vi "ADCP_Raw_Bytes_To_Data_Packet.vi"(8 "error in (no error)":errorcluster, 9 "Raw Packet":u8[](array[numeric]), 10 "Data Packet In":T2, 11 "ADCP in":refnum<class "ADCP.lvclass">) -> (0 "error out":errorcluster, 2 "Data Packet Out":T2, 3 "ADCP out":refnum<class "ADCP.lvclass">)   [LabVIEW 2017, in "ADCP.lvclass"]
uses:
  ADCP.lvclass
  ADCP_Data_Packet_Transmit_Mode.ctl
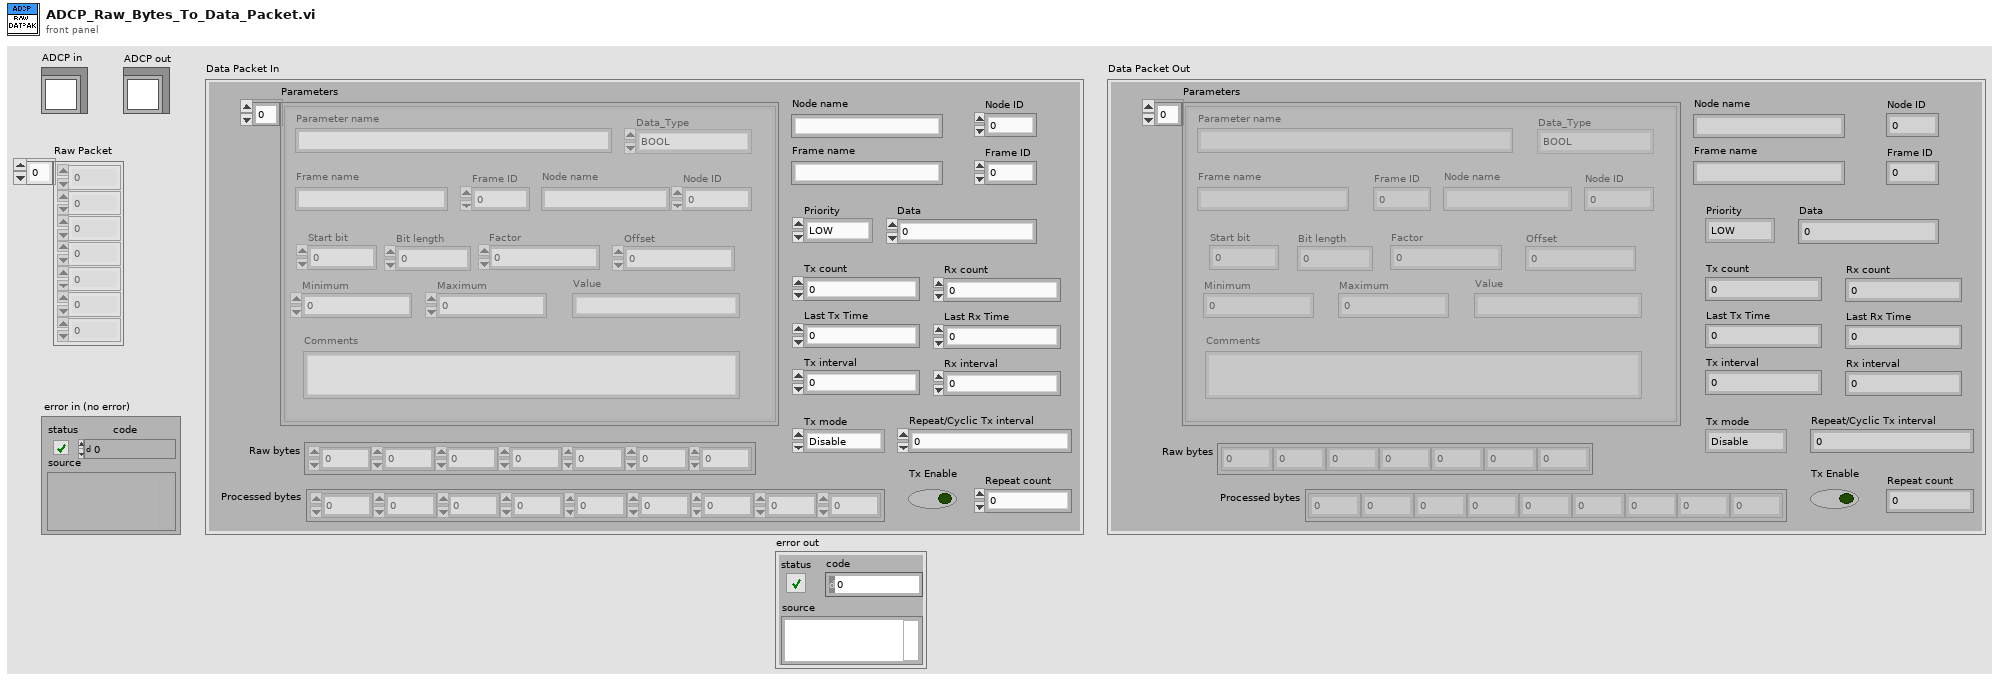
[diagram p1: front panel]
types:
  T1 = typedef "ADCP.lvclass/ADCP_Data_Packet_Transmit_Mode.ctl" = enum16{"Disable", "Single", "Cyclic", "Repeat"}
  T2 = cluster{"Parameters":cluster{"Parameter name":string, "Node name":string, "Node ID":u8, "Frame name":string, "Frame ID":u8, "Start bit":u32, "Bit length":u32, "Factor":dbl, "Offset":dbl, "Minimum":dbl, "Maximum":dbl, "Value":string, "Comments":string, "Data_Type":enum16{"BOOL", "UNSIGNED", "SIGNED", "FLOAT32", "ENUM"}}[], "Priority":enum16{"LOW", "HIGH"}, "Node name":string, "Node ID":u8, "Frame name":string, "Frame ID":u8, "Data":u32, "Raw bytes":u8[], "Processed bytes":u8[], "Tx count":i32, "Last Tx Time":u32, "Tx interval":u32, "Rx count":i32, "Last Rx Time":u32, "Rx interval":u32, "Tx Enable":bool, "Tx mode":T1, "Repeat/Cyclic Tx interval":u32, "Repeat count":u16}
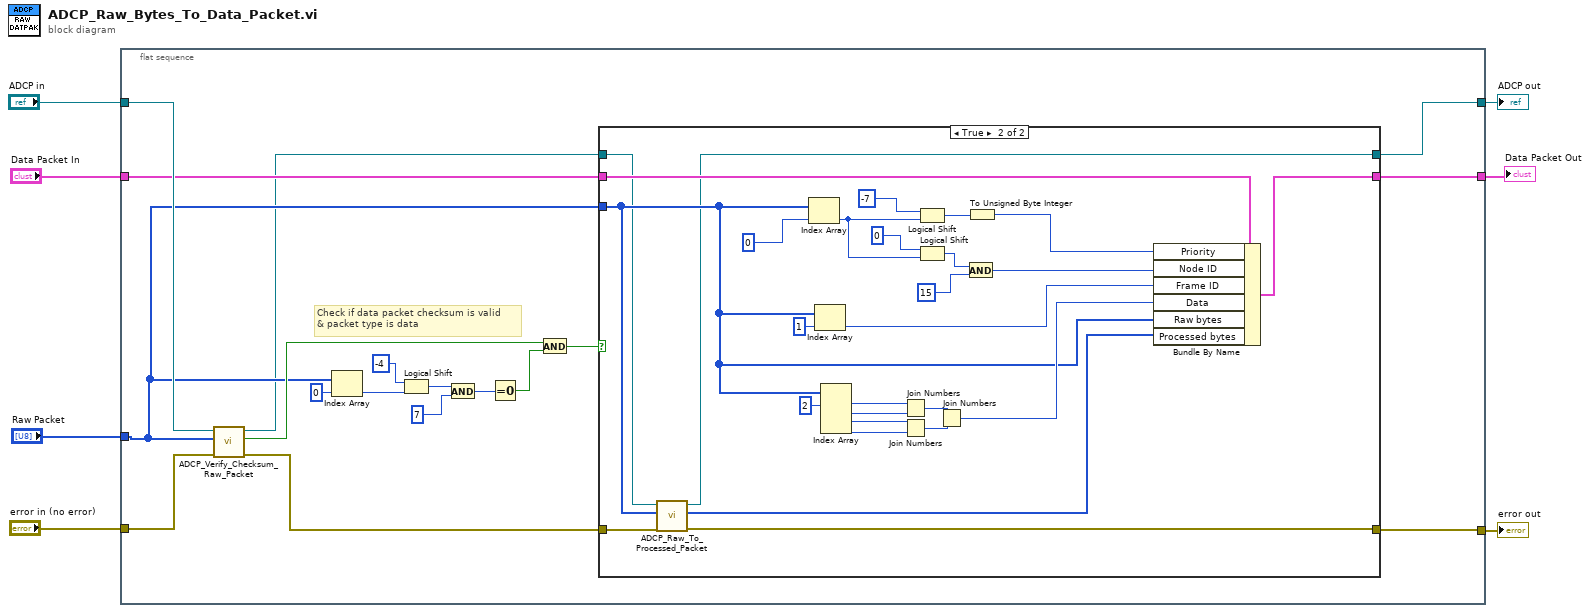
[diagram p0: block diagram]
diagram:
  n1 = flat-sequence {
    tunnel: "ADCP in" -> [w23]
    tunnel: "error in (no error)" -> [w25]
    tunnel: [w8] -> w5
    tunnel: "Raw Packet" -> [w10]
    tunnel: "Data Packet In" -> [w21]
    tunnel: [w22] -> w2
    tunnel: [w20] -> w1
    frame #0 {
      # "Check if data packet checksum is valid\n& packet type is data"
      n2 = call "ADCP_Verify_Checksum_Raw_Packet.vi"("error in (no error)"=w25, "Raw Packet"=w10, "ADCP in"=w23) -> ("error out"=w24:errorcluster, "Checksum Valid ?"=w18:bool, "ADCP out"=w9:refnum<class "ADCP.lvclass">)  [unwired: 6 in]
      n3 = Index Array(array=w10, index=0) -> (element=w16:u8)
      n4 = Logical Shift(y=i16 -4, x=w16) -> (x << y=w14:u8)
      n5 = And(x=w14, y=u8 7) -> (x .and. y?=w12:u8)
      n6 = Equal To 0?(x=w12) -> (x = 0?=w11:bool)
      n7 = And(x=w18, y=w11) -> (x .and. y?=w19:bool)
      n8 = case shown="True" w19 {
        tunnel: w24 -> [w28 w34]
        tunnel: [w28 w30] -> w22
        tunnel: w21 -> [w27 w55]
        tunnel: [w27 w54] -> w20
        tunnel: w10 -> [_ w33]
        tunnel: w9 -> [w26 w32]
        tunnel: [w26 w29] -> w8
        frame False {
        }
        frame True {
          n9 = call "ADCP_Raw_To_Processed_Packet.vi"("error in (no error)"=w34, "Raw Packet"=w33, "ADCP in"=w32) -> ("error out"=w30:errorcluster, "Processed Packet"=w31:u8[], "ADCP out"=w29:refnum<class "ADCP.lvclass">)  [unwired: 6 in]
          n10 = Index Array(array=w33, index=0) -> (element=w49:u8)
          n11 = Index Array(array=w33, index=1) -> (element=w43:u8)
          n12 = Index Array(array=w33, index #1=2 ("index")) -> (element #1=w41:u8, element #2=w40:u8, element #3=w39:u8, element #4=w38:u8)  [unwired: 3 in]
          n13 = Join Numbers(hi=w41, lo=w40) -> ((hi.lo)=w37:u16)
          n14 = Join Numbers(hi=w39, lo=w38) -> ((hi.lo)=w36:u16)
          n15 = Logical Shift(y=i16 -7, x=w49) -> (x << y=w51:u8)
          n16 = Logical Shift(y=i16 0, x=w49) -> (x << y=w47:u8)
          n17 = Join Numbers(hi=w37, lo=w36) -> ((hi.lo)=w35:u32)
          n18 = And(x=w47, y=u8 15) -> (x .and. y?=w45:u8)
          n19 = To Unsigned Byte Integer(number=w51) -> (unsigned 8bit integer=w50:u8)
          n20 = Bundle By Name(cluster=w55, "Priority"=w50, "Node ID"=w45, "Frame ID"=w43, "Data"=w35, "Raw bytes"=w33, "Processed bytes"=w31) -> (w54:T2)
        }
      }
    }
  }
  "ADCP out" <- w5
  "error out" <- w2
  "Data Packet Out" <- w1
